vi "Read_Target_Address.vi"(8 "error in (no error)":errorcluster, 11 "10Bit_Address in":refnum<class "10Bit_Address.lvclass">) -> (0 "error out":errorcluster, 2 "Target_Address":u16 format="%x", 3 "10Bit_Address out":refnum<class "10Bit_Address.lvclass">)   [LabVIEW 2023, in "10Bit_Address.lvclass"]
uses:
  10Bit_Address/10Bit_Address.lvclass
  10Bit_Address/10Bit_Address.lvclass/10Bit_Address.ctl
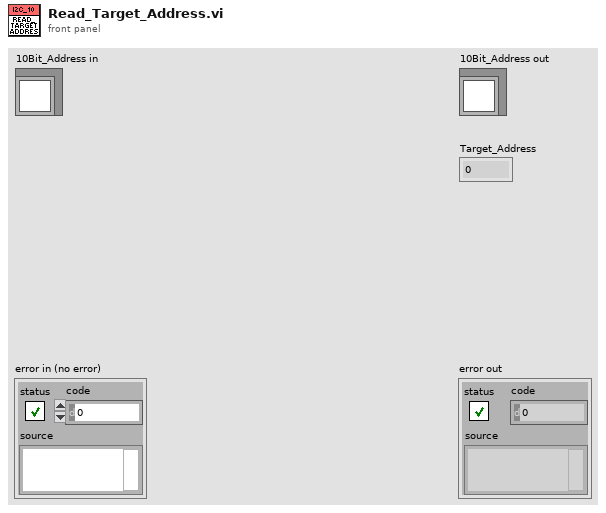
[diagram p1: front panel]
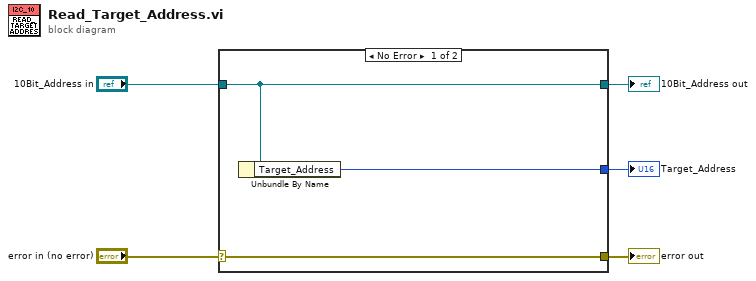
[diagram p0: block diagram]
diagram:
  n1 = case shown="No Error" "error in (no error)" {
    selector: "error in (no error)" -> [w8 w9]
    tunnel: [w8 w9] -> w4
    tunnel: [w7 w10] -> w2
    tunnel: "10Bit_Address in" -> [w7 w10]
    tunnel: [w6 _] -> w1
    frame No Error {
      n2 = Unbundle By Name(w7) -> ("Target_Address"=w6:u16)
    }
    frame Error {
    }
  }
  "error out" <- w4
  "10Bit_Address out" <- w2
  "Target_Address" <- w1
